vi "Colour_codings.vi"() -> ()   [LabVIEW 2010]
panel:
  in  "Optional (informative)":u32(colorbox)=6736896
  in  "Essential input":u32(colorbox)=16776960
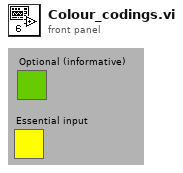
[diagram p1: front panel]
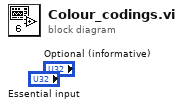
[diagram p0: block diagram]
diagram:
